vi "AMI135Monitor.vi"() -> ()   [LabVIEW 2019]
uses:
  Instrument_Setup.vi
  Global/Global Variables/Data_Display_global.vi
panel:
  out "Helium (%)":dbl
  out "error out":T1
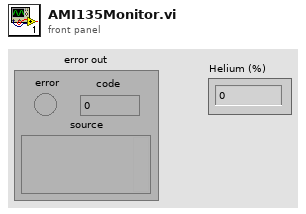
[diagram p1: front panel]
types:
  T1 = cluster{"error":bool, "code":i32, "source":string}
  T2 = cluster{"Sensor Length (cm)":sgl, "Hi Setpoint (cm)":sgl, "Lo Setpoint (cm)":sgl, "Sampling Interval (min)":sgl}
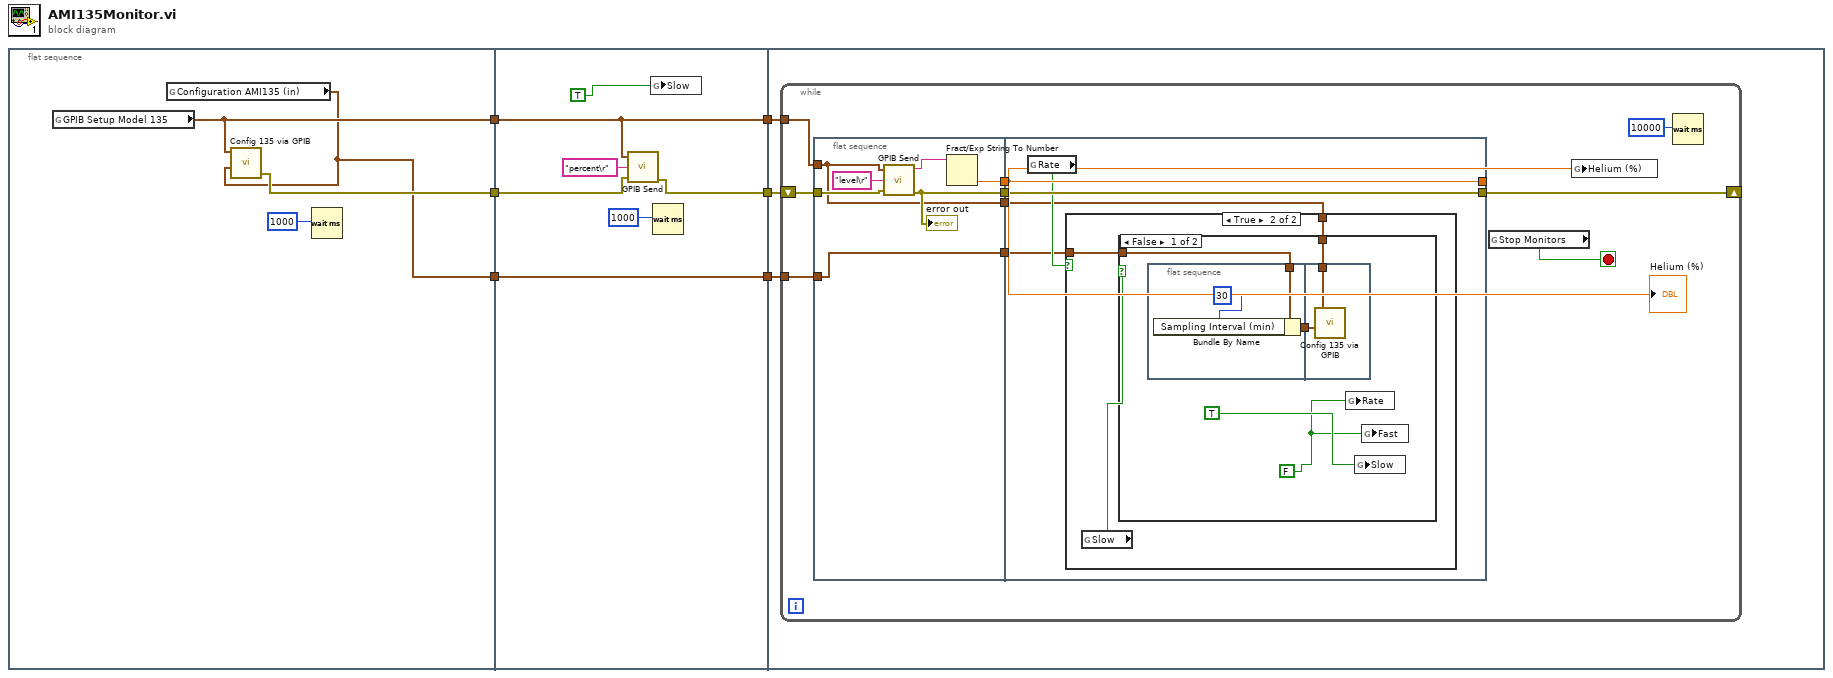
[diagram p0: block diagram]
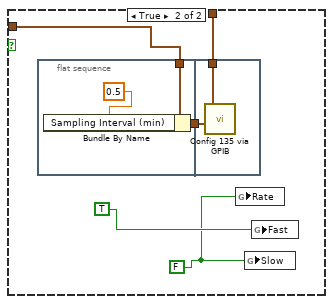
[diagram p3: hidden frame]
diagram:
  n1 = flat-sequence {
    tunnel: [w9] -> w6
    tunnel: [w10] -> w4
    tunnel: [w7] -> w1
    tunnel: w6 -> [w15]
    tunnel: [w14] -> w5
    tunnel: w4 -> [w16]
    tunnel: [w16] -> w3
    tunnel: [w11] -> w2
    tunnel: w1 -> [w11]
    tunnel: w5 -> [w20]
    tunnel: w3 -> [w19]
    tunnel: w2 -> [w18]
    frame #0 {
      n2 = global read "Instrument_Setup.vi" "GPIB Setup Model 135"() -> (w10:cluster{"GPIB address":i16, "GPIB bus":i16})
      n3 = global read "Instrument_Setup.vi" "Configuration AMI135 (in)"() -> (w7:T2)
      n4 = call "Config 135 via GPIB.vi"("Configuration (in)"=w7, "GPIB Setup"=w10) -> ("error out"=w9:T1)  [unwired: 2 in, 2 out]
      n5 = Wait (ms)(milliseconds to wait=1000) -> ()  [unwired: 1 out]
    }
    frame #1 {
      n6 = call "GPIB Send.vi"("GPIB Setup"=w16, "Input command"="percent\r", "error in"=w15) -> ("error out"=w14:T1)  [unwired: 3 out]
      n7 = global write "Data_Display_global.vi" "Slow"(TRUE) -> ()
      n8 = Wait (ms)(milliseconds to wait=1000) -> ()  [unwired: 1 out]
    }
    frame #2 {
      n9 = while {
        shift-right: [w30] -> _
        shift-left: w20 -> [w27]
        tunnel: w19 -> [w28]
        tunnel: w18 -> [w22]
        stop <- w29 stop-if-true
        n10 = flat-sequence {
          tunnel: w28 -> [w32]
          tunnel: w27 -> [w35]
          tunnel: [w37] -> w25
          tunnel: [w36] -> w24
          tunnel: [w33] -> w23
          tunnel: w22 -> [w33]
          tunnel: [w32] -> w21
          tunnel: [w42] -> w30
          tunnel: [w43] -> w31
          tunnel: w25 -> [w43]
          tunnel: w24 -> [w42]
          tunnel: w23 -> [w40]
          tunnel: w21 -> [w39]
          frame #0 {
            n11 = call "GPIB Send.vi"("GPIB Setup"=w32, "Input command"="level\r", "error in"=w35) -> ("Return string"=w34:string, "error out"=w36:T1)  [unwired: 2 out]
            "error out" <- w36
            n12 = Fract/Exp String To Number(string=w34) -> (number=w37:dbl)  [unwired: 3 in, 1 out]
          }
          frame #1 {
            n13 = global read "Data_Display_global.vi" "Rate"() -> (w41:bool)
            n14 = case shown="True" w41 {
              tunnel: w40 -> [_ w45]
              tunnel: w39 -> [_ w44]
              frame False {
              }
              frame True {
                n15 = global read "Data_Display_global.vi" "Slow"() -> (w46:bool)
                n16 = case shown="False" w46 {
                  tunnel: w45 -> [w50 w61]
                  tunnel: w44 -> [w49 w59]
                  frame False {
                    w47 = FALSE
                    n17 = flat-sequence {
                      tunnel: w50 -> [w53]
                      tunnel: [w52] -> w51
                      tunnel: w51 -> [w56]
                      tunnel: w49 -> [w55]
                      frame #0 {
                        n18 = Bundle By Name(cluster=w53, "Sampling Interval (min)"=30) -> (w52:T2)
                      }
                      frame #1 {
                        n19 = call "Config 135 via GPIB.vi"("Configuration (in)"=w56, "GPIB Setup"=w55) -> ()  [unwired: 2 in, 3 out]
                      }
                    }
                    n20 = global write "Data_Display_global.vi" "Rate"(w47) -> ()
                    n21 = global write "Data_Display_global.vi" "Slow"(TRUE) -> ()
                    n22 = global write "Data_Display_global.vi" "Fast"(w47) -> ()
                  }
                  frame True {
                    w57 = FALSE
                    n23 = flat-sequence {
                      tunnel: w61 -> [w63]
                      tunnel: [w62] -> w60
                      tunnel: w60 -> [w66]
                      tunnel: w59 -> [w65]
                      frame #0 {
                        n24 = Bundle By Name(cluster=w63, "Sampling Interval (min)"=0.5) -> (w62:T2)
                      }
                      frame #1 {
                        n25 = call "Config 135 via GPIB.vi"("Configuration (in)"=w66, "GPIB Setup"=w65) -> ()  [unwired: 2 in, 3 out]
                      }
                    }
                    n26 = global write "Data_Display_global.vi" "Rate"(w57) -> ()
                    n27 = global write "Data_Display_global.vi" "Slow"(w57) -> ()
                    n28 = global write "Data_Display_global.vi" "Fast"(TRUE) -> ()
                  }
                }
              }
            }
          }
        }
        n29 = global read "Data_Display_global.vi" "Stop Monitors"() -> (w29:bool)
        n30 = global write "Data_Display_global.vi" "Helium (%)"(w31) -> ()
        n31 = Wait (ms)(milliseconds to wait=10000) -> ()  [unwired: 1 out]
        "Helium (%)" <- w31
      }
    }
  }
